vi "Draw_ROI.vi"(6 "Color":u32, 9 "클러스터":cluster{dbl, dbl}, 10 "Group":string, 11 "참조 번호 입력":T1) -> (3 "참조 번호 출력":T1)   [LabVIEW 2014]
uses:
  <vilib>/vision/Image Controls.llb/IMAQ Image.ctl
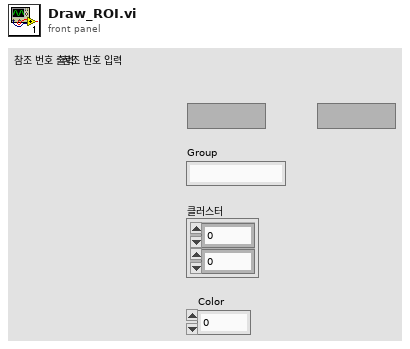
[diagram p1: front panel]
types:
  T1 = typedef "IMAQ Image.ctl" = refnum<image>
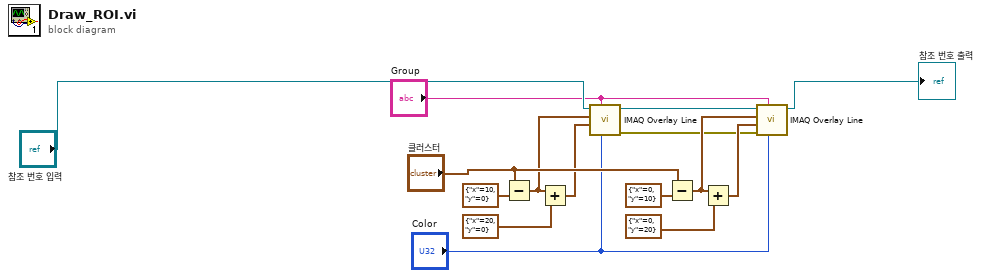
[diagram p0: block diagram]
diagram:
  n1 = Subtract(x="클러스터", y=cluster{"x":i32, "y":i32} {"x"=10, "y"=0}) -> (x-y=w9:cluster{dbl, dbl})
  n2 = Add(x=w9, y=cluster{"x":i32, "y":i32} {"x"=20, "y"=0}) -> (x+y=w7:cluster{dbl, dbl})
  n3 = call "IMAQ Overlay Line"("Color"="Color", "Group"="Group", "End Point"=w7, "Start Point"=w9, "Image"="참조 번호 입력") -> ("error out"=w1:errorcluster, "Image Out"=w2:T1)  [unwired: 1 in, 4 out]
  n4 = Subtract(x="클러스터", y=cluster{"x":i32, "y":i32} {"x"=0, "y"=10}) -> (x-y=w5:cluster{dbl, dbl})
  n5 = Add(x=w5, y=cluster{"x":i32, "y":i32} {"x"=0, "y"=20}) -> (x+y=w6:cluster{dbl, dbl})
  n6 = call "IMAQ Overlay Line"("Color"="Color", "Group"="Group", "error in (no error)"=w1, "End Point"=w6, "Start Point"=w5, "Image"=w2) -> ("Image Out"=→"참조 번호 출력":T1)  [unwired: 5 out]
